vi "AllowTDCFastRead.vi"() -> ()   [LabVIEW 2016]
panel:
  out "AllowTDCFastRead":bool
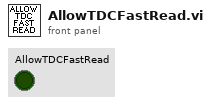
[diagram p1: front panel]
diagram:
